vi "CSV Save.vi"(9 "Array":dbl[][](array[numeric]), 11 "Save Button":bool caption="Save Process") -> (3 "Save Status":bool)   [LabVIEW 2018]
uses:
  <vilib>/Utility/file.llb/Write To Spreadsheet File (DBL).vi
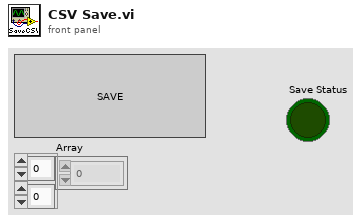
[diagram p1: front panel]
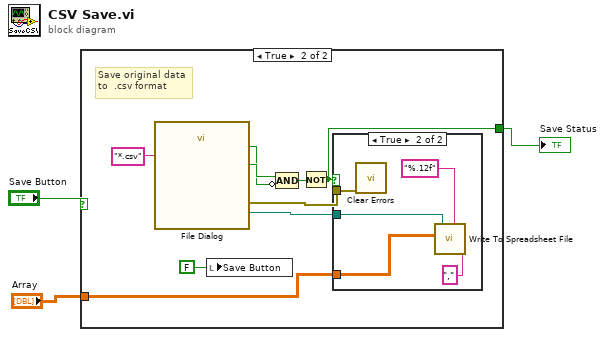
[diagram p0: block diagram]
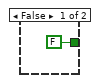
[diagram p2: hidden frame]
diagram:
  n1 = case shown="True" "Save Button" {
    tunnel: "Array" -> [_ w13]
    tunnel: [FALSE w5] -> w1
    frame False {
    }
    frame True {
      # "Save original data\nto  .csv format"
      n2 = call "File Dialog"("pattern (all files)"="*.csv") -> ("selected path"=w11:path, "exists"=w9:bool, "cancelled"=w10:bool, "error out"=w8:errorcluster)  [unwired: 11 in]
      n3 = local write "Save Button"(FALSE ("Save Button")) -> ()
      n4 = Compound Arithmetic op=AND(w10, invert w9) -> (w6:bool)
      n5 = Not(x=w6) -> (.not. x?=w5:bool)
      n6 = case shown="True" w5 {
        tunnel: w13 -> [_ w18]
        tunnel: w11 -> [_ w16]
        tunnel: w8 -> [_ w14]
        frame False {
        }
        frame True {
          n7 = call <vilib>:"Clear Errors.vi"("error in (no error)"=w14) -> ()  [unwired: 5 in, 2 out]
          n8 = call-poly <vilib>:"Write To Spreadsheet File.vi"("delimiter (\\t)"="," ("delimiter (\\t)"), "format (%.3f)"="%.12f", "2D data"=w18, "file path (dialog if empty)"=w16) -> ()  [unwired: 4 in, 1 out]
        }
      }
    }
  }
  "Save Status" <- w1
